vi "MSScript_SubVI_ArrayIndice.vi"(9 "@name[x:y|z]":string="@Array[$abc]") -> (0 "Index no found":bool, 2 "Indice string":string, 3 "@name":string)   [LabVIEW 2018, in "MSScript.lvclass"]
uses:
  MSScript.lvclass
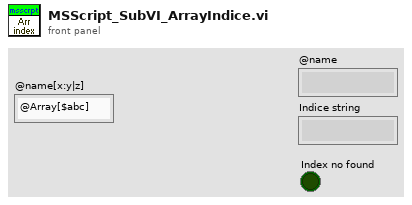
[diagram p1: front panel]
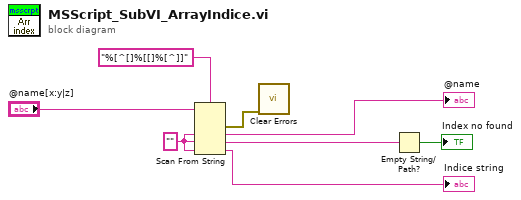
[diagram p0: block diagram]
diagram:
  w6 = "" ("format string")
  n1 = Scan From String(format string="%[^[]%[[]%[^]]", input string="@name[x:y|z]", default 1=w6, default 2=w6, default 3=w6) -> (error out=w3:errorcluster, output 1=→"@name":string, output 2=w4:string, output 3=→"Indice string":string)  [unwired: 2 in, 2 out]
  n2 = call <vilib>:"Clear Errors.vi"("error in (no error)"=w3) -> ()  [unwired: 5 in, 2 out]
  n3 = Empty String/Path?(string/path=w4) -> (empty?=→"Index no found":bool)
